vi "GetHelp.vi"(11 "SecureRunVI in":refnum<class "SecureRunVI.lvclass">) -> (2 "Help":string, 3 "SecureRunVI out":refnum<class "SecureRunVI.lvclass">)   [LabVIEW 2020, in "SecureRunVI.lvclass"]
doc: "The help message for this operation in the LabVIEWCLI."
uses:
  SecureRunVI.lvclass
panel:
  in  "HelpText":string="LabVIEWCLI -OperationName SecureRunVI -VIPath <path of the vi to run>\n\n -VIPath : Path of the VI to run. For the connector pane of this VI, please refer to how to use document for the RunVI operation.\n"
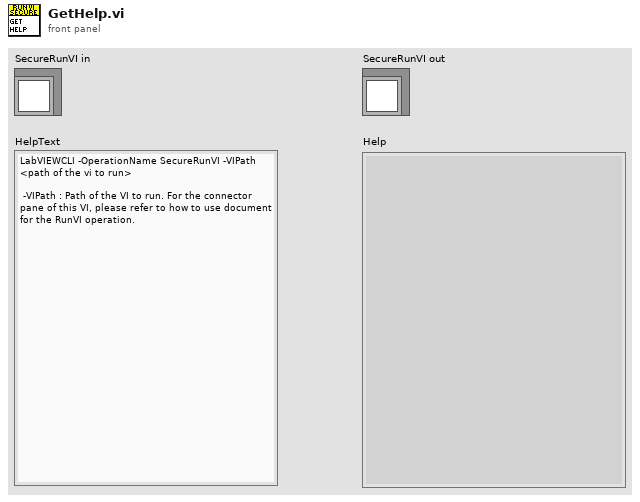
[diagram p1: front panel]
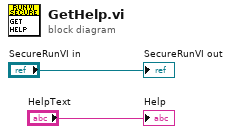
[diagram p0: block diagram]
diagram:
  "SecureRunVI out" <- "SecureRunVI in"
  "Help" <- "HelpText"
